vi "Retry RUN.vi"(8 "error in (no error)":errorcluster, 10 "Next?":bool=TRUE, 11 "Run Block in":refnum<class "Run Block.lvclass">) -> (0 "error out":errorcluster, 3 "Run Block out":refnum<class "Run Block.lvclass">)   [LabVIEW 2020, in "CIRCUS_uServices.lvlib" / "Run Utilities.lvlib" / "Run Block.lvclass"]
doc: "Inerts the Current RUN back into the Schedule"
uses:
  Run Block.lvclass
  Run Block.lvclass/Run Block.ctl
  Schedule/Schedule.lvclass
  Run Instance/Run Instance.lvclass
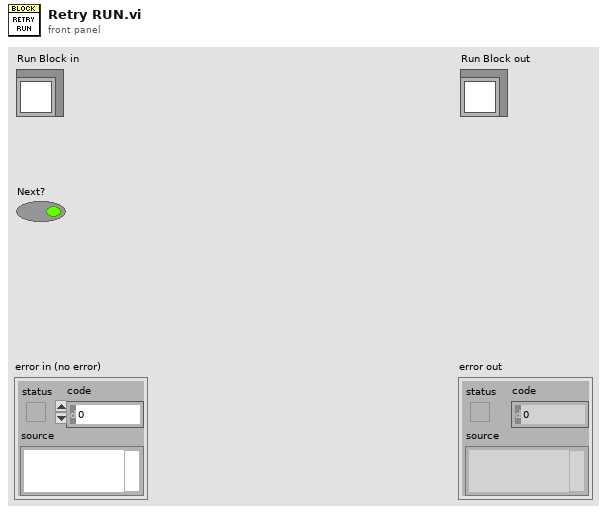
[diagram p1: front panel]
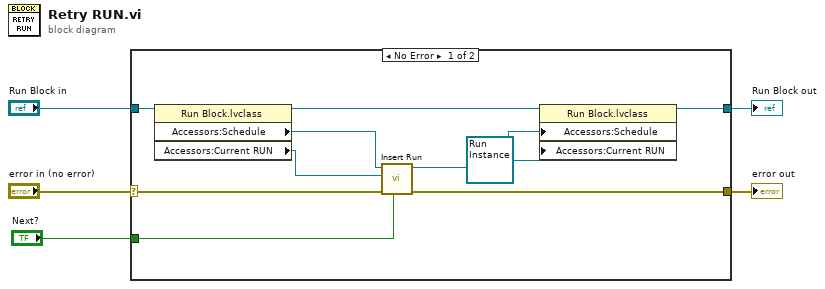
[diagram p0: block diagram]
diagram:
  n1 = case shown="No Error" "error in (no error)" {
    selector: "error in (no error)" -> [w9 w17]
    tunnel: [w8 w17] -> w4
    tunnel: [w13 w16] -> w2
    tunnel: "Run Block in" -> [w15 w16]
    tunnel: "Next?" -> [w7 _]
    frame No Error {
      n2 = property class="Run Block.lvclass"(reference=w15) -> (reference out=w14:refnum<class "Run Block.lvclass">, "Accessors:Schedule"=w12:refnum<class "Schedule.lvclass">, "Accessors:Current RUN"=w11:refnum<class "Run Instance.lvclass">)  [unwired: 1 in, 1 out]
      n3 = call-dynamic "Insert Run.vi"("Reinsert?"=w7, "error in (no error)"=w9, "Run Instance"=w11, "Schedule in"=w12) -> ("error out"=w8:errorcluster, "Schedule out"=w10:refnum<class "Schedule.lvclass">)  [unwired: 5 in, 1 out]
      n4 = property class="Run Block.lvclass"(reference=w14, "Accessors:Schedule"=w10, "Accessors:Current RUN"=refnum<class "Run Instance.lvclass"> refnum ("Current RUN")) -> (reference out=w13:refnum<class "Run Block.lvclass">)  [unwired: 1 in, 1 out]
    }
    frame Error {
    }
  }
  "error out" <- w4
  "Run Block out" <- w2
